vi "Configuration 1.0 JSON Unflatten.vi"(8 "error in (no error)":errorcluster, 11 "dsf configuration json":string) -> (0 "error out":errorcluster, 2 "dsf version":T2, 3 "framework configuration 1.0":T1)   [LabVIEW 2020, in "DSF Core.lvlib" / "Configuration Session.lvclass"]
uses:
  Configuration Session.lvclass
  Typedefs/DSF Version Info.ctl
  DSF Core.lvlib
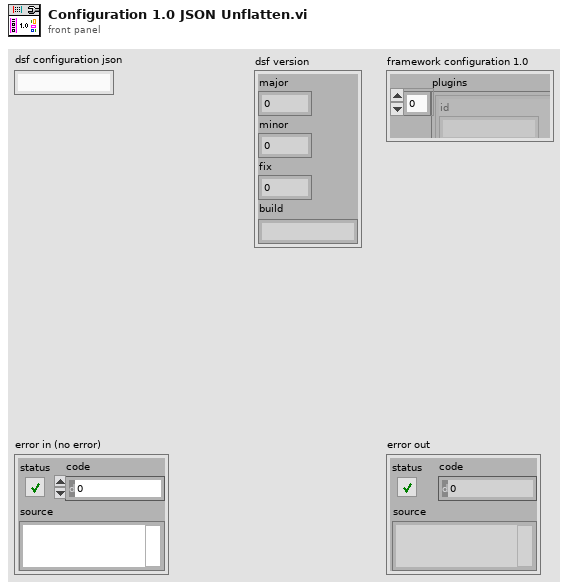
[diagram p1: front panel]
types:
  T1 = cluster{"plugins":cluster{"id":string, "values":cluster{"components":string[], "timing":cluster{"priority":u64, "decimation":u64, "offset":u64}, "group ids":string[], "settings id":string, "threads":cluster{"buffer converter settings":cluster{"key":string, "value":string}[], "transceiver settings":cluster{"key":string, "value":string}[], "custom settings":cluster{"key":string, "value":string}[], "processor":i32, "priority offset":i16}[]}}[], "groups":cluster{"id":string, "values":cluster{"direction":i32, "timing":cluster{"priority":u64, "decimation":u64, "offset":u64}, "transfer ids":string[], "settings id":string, "thread":i32, "timeout behavior":u8}}[], "transfers":cluster{"id":string, "values":cluster{"byte order":i32, "channel ids":string[], "settings id":string}}[], "channels":cluster{"id":string, "values":cluster{"string buffer offset":u64, "string data type":i32, "engine data type":i32, "settings id":string, "units":string}}[], "settings":cluster{"id":string, "values":cluster{"key":string, "value":string}[]}[]}
  T2 = typedef "DSF Core.lvlib/DSF Version Info.ctl" = cluster{"major":u32, "minor":u32, "fix":u32, "build":string}
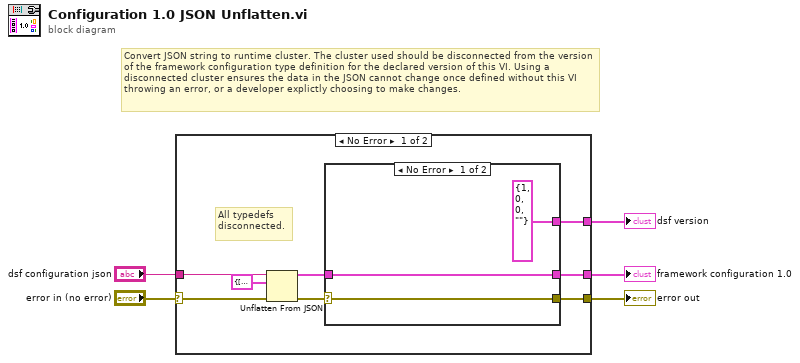
[diagram p0: block diagram]
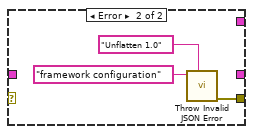
[diagram p2: hidden frame]
diagram:
  # "Convert JSON string to runtime cluster. The cluster used should be disconnected from the version of the framework configuration type definition for the declared version of this VI. Using a disconnected cluster ensures the data in the JSON cannot change once defined without this VI throwing an error, or a developer explictly choosing to make changes."
  n1 = case shown="No Error" "error in (no error)" {
    selector: "error in (no error)" -> [w9 w20]
    tunnel: [w12 w20] -> w5
    tunnel: [w10 _] -> w2
    tunnel: [w8 _] -> w3
    tunnel: "dsf configuration json" -> [w6 _]
    frame No Error {
      # "All typedefs disconnected."
      n2 = Unflatten From JSON(JSON string=w6, type and defaults=T1 {"plugins"=[], "groups"=[], "transfers"=[], "channels"=[], "settings"=[]} ("framework configuration 1.0"), error in (no error)=w9) -> (value=w11:T1, error out=w13:errorcluster)  [unwired: 4 in]
      n3 = case shown="No Error" w13 {
        selector: w13 -> [w16 _]
        tunnel: [w16 w19] -> w12
        tunnel: w11 -> [w14 _]
        tunnel: [w14 _] -> w10
        tunnel: [T2 {"major"=1, "minor"=0, "fix"=0, "build"=""} ("dsf version") _] -> w8
        frame No Error {
        }
        frame Error {
          n4 = call "Throw Invalid JSON Error.vi"("error source vi name"="Unflatten 1.0", "name"="framework configuration") -> ("error out"=w19:errorcluster)  [unwired: 9 in]
        }
      }
    }
    frame Error {
    }
  }
  "error out" <- w5
  "dsf version" <- w3
  "framework configuration 1.0" <- w2
